vi "Create Rx.vi"(8 "error in (no error)":errorcluster, 10 "Reader Name":string, 11 "RxTx in":refnum<class "RxTx.lvclass">) -> (0 "error out":errorcluster, 3 "RxTx out":refnum<class "RxTx.lvclass">)   [LabVIEW 2018, in "RxTx.lvclass"]
uses:
  RxTx.lvclass
  RxTx.lvclass/RxTx.ctl
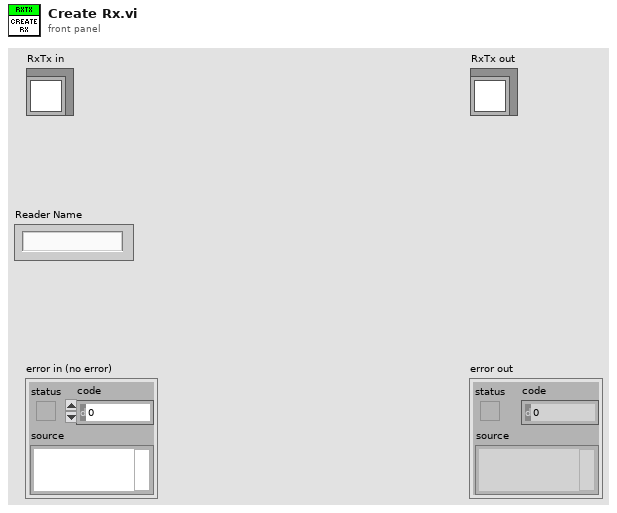
[diagram p1: front panel]
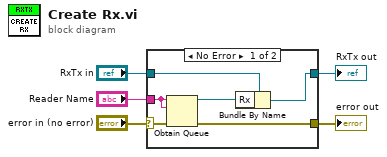
[diagram p0: block diagram]
diagram:
  n1 = case shown="No Error" "error in (no error)" {
    selector: "error in (no error)" -> [w10 w13]
    tunnel: [w11 w13] -> w4
    tunnel: [w7 w12] -> w2
    tunnel: "RxTx in" -> [w8 w12]
    tunnel: "Reader Name" -> [w9 _]
    frame No Error {
      n2 = Obtain Queue(name (unnamed)=w9, element data type=w9, error in (no error)=w10) -> (queue out=w6:refnum<queue>, error out=w11:errorcluster)  [unwired: 2 in, 1 out]
      n3 = Bundle By Name(cluster=w8, "Rx"=w6) -> (w7:refnum<class "RxTx.lvclass">)
    }
    frame Error {
    }
  }
  "error out" <- w4
  "RxTx out" <- w2
